vi "单个均值化.vi"(1 "温度信号 4":waveform(dbl)(graph), 2 "传感器灵敏度":dbl=1.0) -> (0 "温度信号 3":waveform(dbl)(graph))   [LabVIEW 2014]
panel:
  out "元素":i32
  out "大小":i32[](array[numeric])
  out "Array":dbl[][](array[numeric]) caption="数组"
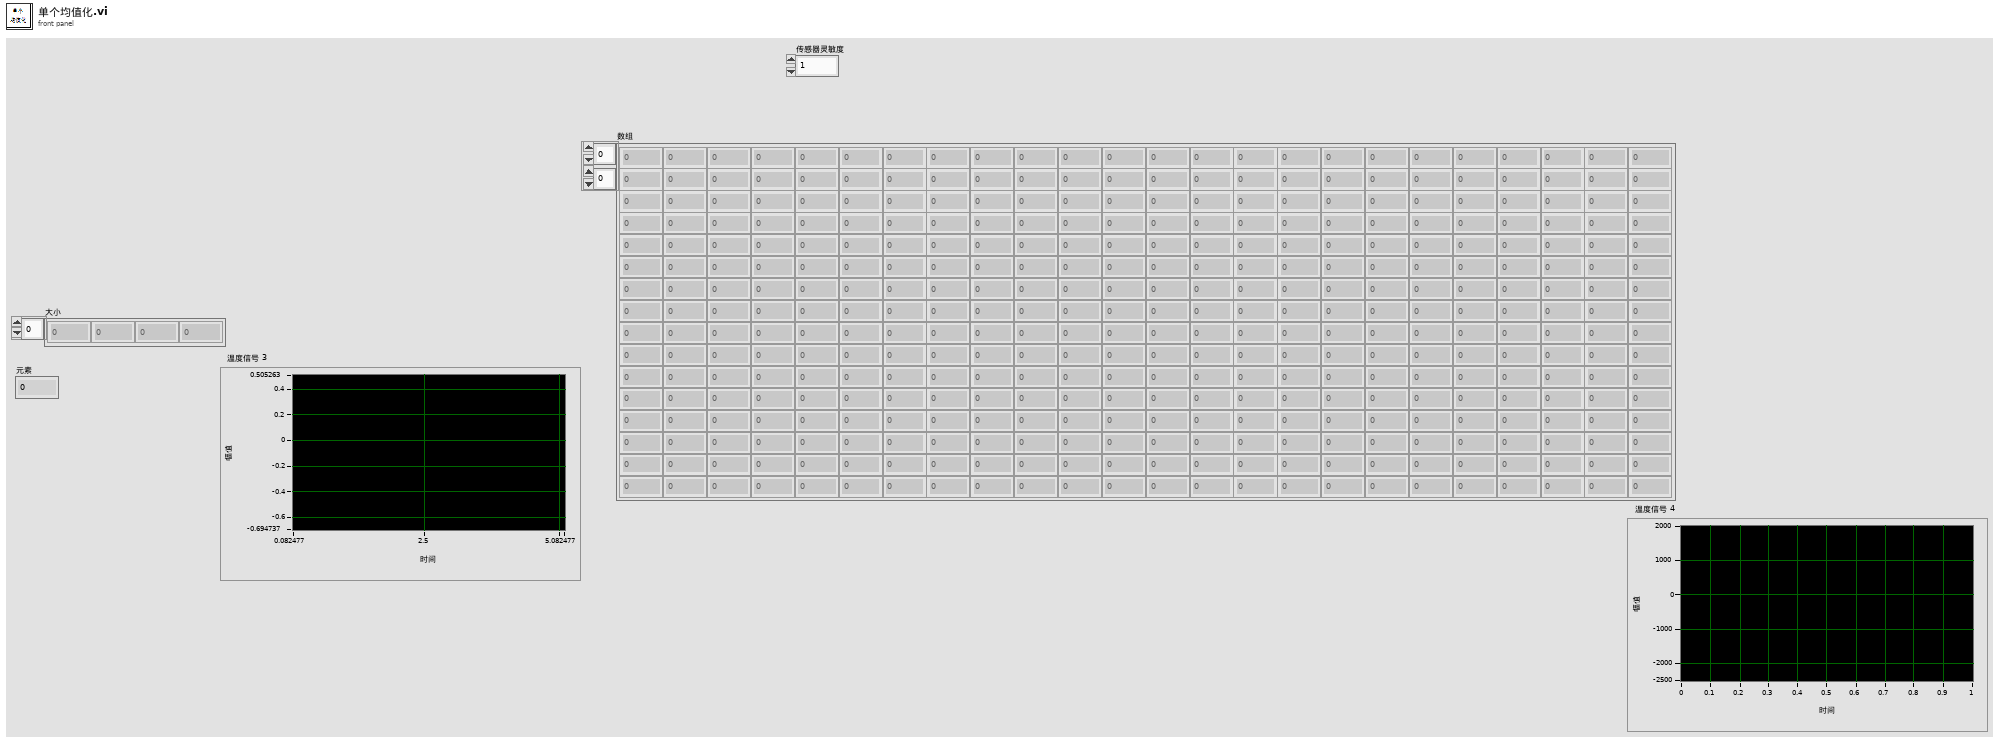
[diagram p1: front panel]
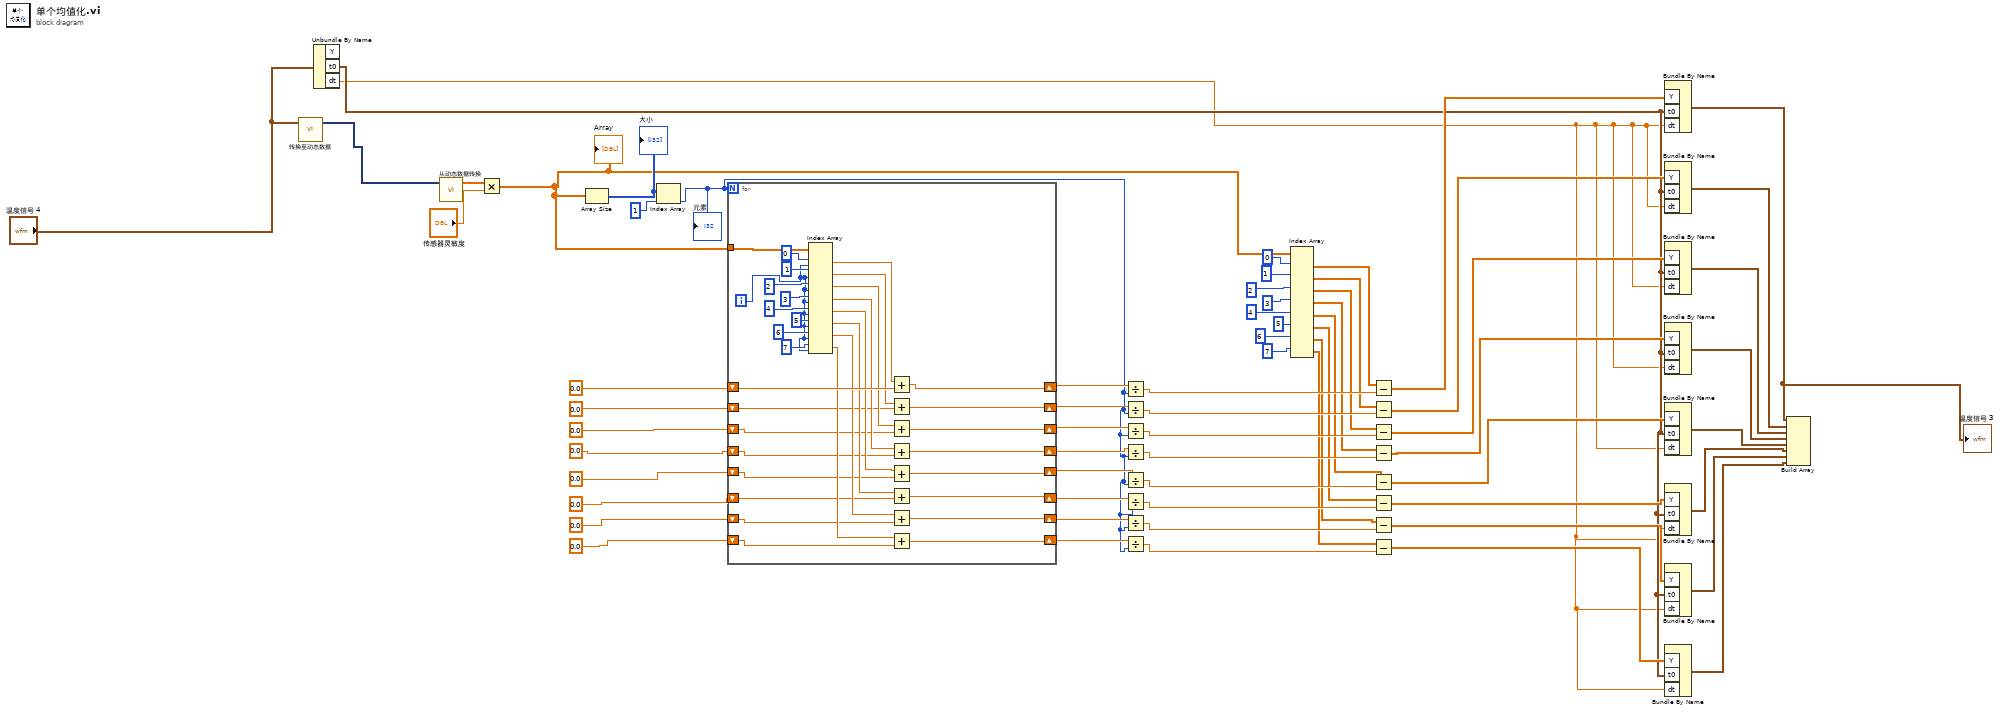
[diagram p0: block diagram]
diagram:
  n1 = call "转换至动态数据"("Waveform"="温度信号 4") -> ("Dynamic Data Type"=w3:dynamicdata)  [unwired: 3 in]
  n2 = Unbundle By Name("温度信号 4") -> ("t0"=w12:timestamp, "dt"=w11:dbl)  [unwired: 1 out]
  n3 = call "从动态数据转换"("Dynamic Data Type"=w3) -> ("Array"=w23:dbl[][])  [unwired: 3 in]
  n4 = Multiply(x=w23, y="传感器灵敏度") -> (x*y=w21:dbl[][])
  "Array" <- w21
  n5 = Array Size(array=w21) -> (size(s)=w26:i32[])
  "大小" <- w26
  n6 = Index Array(array=w26, index=1) -> (element=w25:i32)
  "元素" <- w25
  n7 = for {
    N: w25 -> [_]
    tunnel: w21 -> [w98]
    shift-right: [w74] -> w58
    shift-left: 0.0 -> [w90]
    shift-right: [w73] -> w57
    shift-left: 0.0 -> [w81]
    shift-right: [w72] -> w56
    shift-left: 0.0 -> [w80]
    shift-right: [w71] -> w55
    shift-left: 0.0 -> [w79]
    shift-right: [w70] -> w54
    shift-left: 0.0 -> [w78]
    shift-right: [w69] -> w53
    shift-left: 0.0 -> [w77]
    shift-right: [w68] -> w52
    shift-left: 0.0 -> [w76]
    shift-right: [w67] -> w51
    shift-left: 0.0 -> [w75]
    i -> [w91]
    n8 = Index Array(array=w98, index (row) #1=0 ("索引 (行)"), index (col) #1=w91, index (row) #2=1 ("索引 (行)"), index (col) #2=w91, index (row) #3=2 ("索引 (行)"), index (col) #3=w91, index (row) #4=3 ("索引 (行)"), index (col) #4=w91, index (row) #5=4 ("索引 (行)"), index (col) #5=w91, index (row) #6=5 ("索引 (行)"), index (col) #6=w91, index (row) #7=6 ("索引 (行)"), index (col) #7=w91, index (row) #8=7 ("索引 (行)"), index (col) #8=w91) -> (element #1=w89:dbl, element #2=w88:dbl, element #3=w87:dbl, element #4=w86:dbl, element #5=w85:dbl, element #6=w84:dbl, element #7=w83:dbl, element #8=w82:dbl)
    n9 = Add(x=w89, y=w90) -> (x+y=w74:dbl)
    n10 = Add(x=w88, y=w81) -> (x+y=w73:dbl)
    n11 = Add(x=w87, y=w80) -> (x+y=w72:dbl)
    n12 = Add(x=w86, y=w79) -> (x+y=w71:dbl)
    n13 = Add(x=w85, y=w78) -> (x+y=w70:dbl)
    n14 = Add(x=w84, y=w77) -> (x+y=w69:dbl)
    n15 = Add(x=w83, y=w76) -> (x+y=w68:dbl)
    n16 = Add(x=w82, y=w75) -> (x+y=w67:dbl)
  }
  n17 = Divide(x=w58, y=w25) -> (x/y=w42:dbl)
  n18 = Divide(x=w57, y=w25) -> (x/y=w41:dbl)
  n19 = Divide(x=w56, y=w25) -> (x/y=w40:dbl)
  n20 = Divide(x=w55, y=w25) -> (x/y=w39:dbl)
  n21 = Divide(x=w54, y=w25) -> (x/y=w38:dbl)
  n22 = Divide(x=w53, y=w25) -> (x/y=w37:dbl)
  n23 = Divide(x=w52, y=w25) -> (x/y=w36:dbl)
  n24 = Divide(x=w51, y=w25) -> (x/y=w35:dbl)
  n25 = Index Array(array=w21, index (row) #1=0 ("索引 (行)"), index (row) #2=1 ("索引 (行)"), index (row) #3=2 ("索引 (行)"), index (row) #4=3 ("索引 (行)"), index (row) #5=4 ("索引 (行)"), index (row) #6=5 ("索引 (行)"), index (row) #7=6 ("索引 (行)"), index (row) #8=7 ("索引 (行)")) -> (element #1=w34:dbl[], element #2=w33:dbl[], element #3=w32:dbl[], element #4=w31:dbl[], element #5=w30:dbl[], element #6=w29:dbl[], element #7=w28:dbl[], element #8=w27:dbl[])  [unwired: 8 in]
  n26 = Subtract(x=w34, y=w42) -> (x-y=w20:dbl[])
  n27 = Subtract(x=w33, y=w41) -> (x-y=w19:dbl[])
  n28 = Subtract(x=w32, y=w40) -> (x-y=w18:dbl[])
  n29 = Subtract(x=w31, y=w39) -> (x-y=w17:dbl[])
  n30 = Subtract(x=w30, y=w38) -> (x-y=w16:dbl[])
  n31 = Subtract(x=w29, y=w37) -> (x-y=w15:dbl[])
  n32 = Subtract(x=w28, y=w36) -> (x-y=w14:dbl[])
  n33 = Subtract(x=w27, y=w35) -> (x-y=w13:dbl[])
  n34 = Bundle By Name("Y"=w20, "t0"=w12, "dt"=w11) -> (w2:waveform(dbl))  [unwired: 1 in]
  "温度信号 3" <- w2
  n35 = Bundle By Name("Y"=w19, "t0"=w12, "dt"=w11) -> (w10:waveform(dbl))  [unwired: 1 in]
  n36 = Bundle By Name("Y"=w18, "t0"=w12, "dt"=w11) -> (w9:waveform(dbl))  [unwired: 1 in]
  n37 = Bundle By Name("Y"=w17, "t0"=w12, "dt"=w11) -> (w8:waveform(dbl))  [unwired: 1 in]
  n38 = Bundle By Name("Y"=w16, "t0"=w12, "dt"=w11) -> (w7:waveform(dbl))  [unwired: 1 in]
  n39 = Bundle By Name("Y"=w15, "t0"=w12, "dt"=w11) -> (w6:waveform(dbl))  [unwired: 1 in]
  n40 = Bundle By Name("Y"=w14, "t0"=w12, "dt"=w11) -> (w5:waveform(dbl))  [unwired: 1 in]
  n41 = Bundle By Name("Y"=w13, "t0"=w12, "dt"=w11) -> (w4:waveform(dbl))  [unwired: 1 in]
  n42 = Build Array(w2, w10, w9, w8, w7, w6, w5, w4) -> ()  [unwired: 1 out]
